vi "Test DeviceManager API.vi"() -> ()   [LabVIEW 2023, in "DeviceManager.lvlib"]
doc: "DeviceManager API Tester."
uses:
  DeviceManager.lvlib
  <vilib>/Utility/error.llb/DialogType.ctl
  2ec88339-7153-484d-8eb7-3b0f2fceeaf8.vi
  SCD/SCD.lvclass
  Mono/Monochromator.lvclass
  CCD/CCD.lvclass
  <vilib>/JDP Science/JSONtext/Variant to JSON Text.vi
  <vilib>/JDP Science/JSONtext/LVClass Serializer/JSONtext LVClass Serializer.lvclass
  <vilib>/Hampel Software Engineering/HSE Logger/hse-logger.lvlib
panel:
  in  "DevicesList":bool
  in  "DiscoverDevices":bool
  in  "JSON to be sent":string="{\"id\":1234, \"command\":\"icl_info\"}"
  in  "SendJSONandAskForReply":bool
  in  "ICLshutdown":bool
  in  "WS Server Port":string="25010"
  in  "WS Server IP":string="ws://127.0.0.1"
  in  "OpenWebSocketCommunication":bool
  in  "StartICL":bool
  out "last error":errorcluster
  in  "Show Diagram on Init":bool
  in  "Show Block Diagram":bool
  in  "Stop Module":bool
  in  "Start Module":bool
  in  "Hide Module Panel":bool
  in  "Show Module Panel":bool
  out "Status":string
  out "Module Running?":bool
  # "This VI tests the API for the Module."
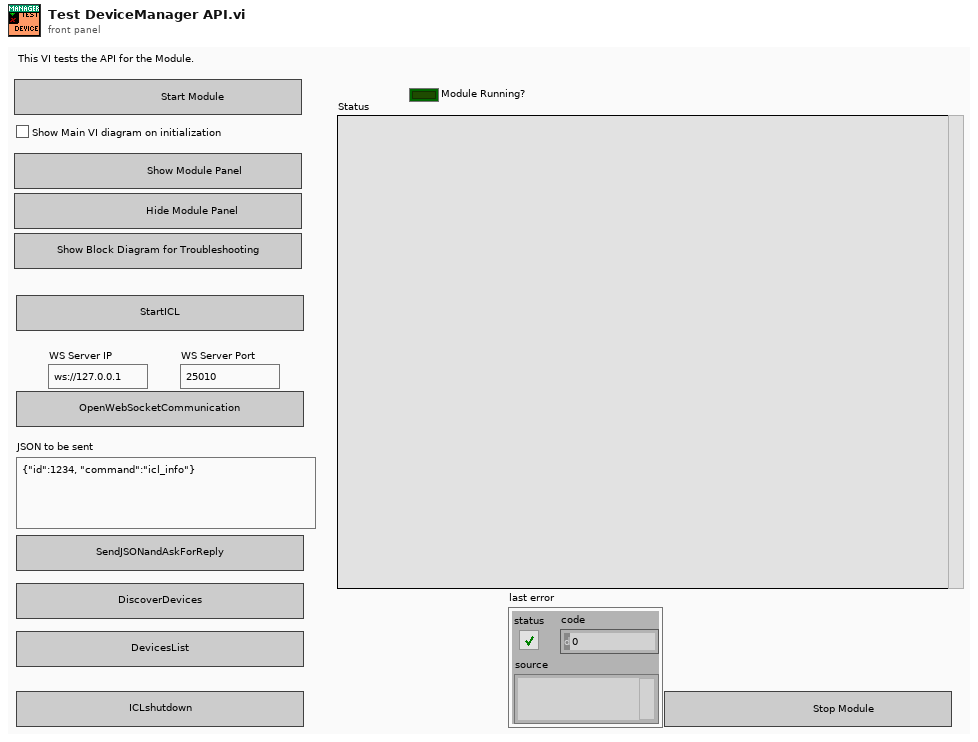
[diagram p1: front panel]
types:
  T1 = typedef "DeviceManager.lvlib/Broadcast Events--cluster.ctl" = cluster{"Module Did Init":refnum<user-event>, "Status Updated":refnum<user-event>, "Error Reported":refnum<user-event>, "Module Did Stop":refnum<user-event>, "Update Module Execution Status":refnum<user-event>}
  T2 = typedef "DialogType.ctl" = u16
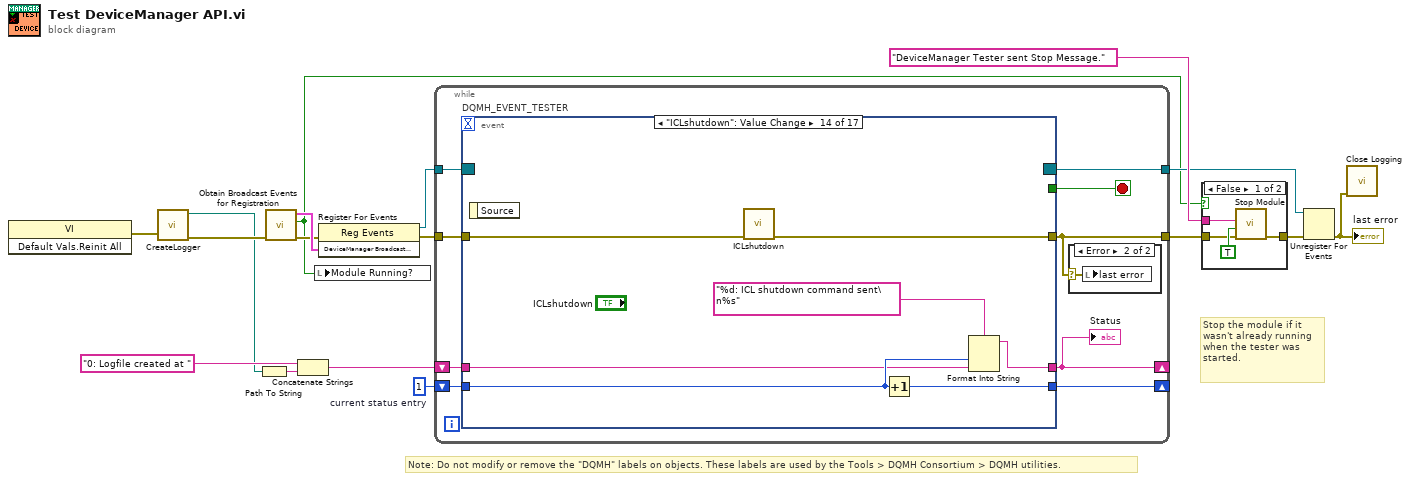
[diagram p0: block diagram]
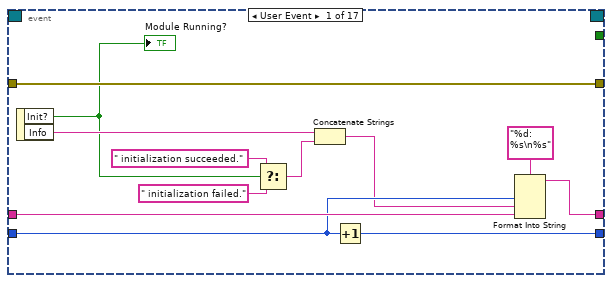
[diagram p4: hidden frame]
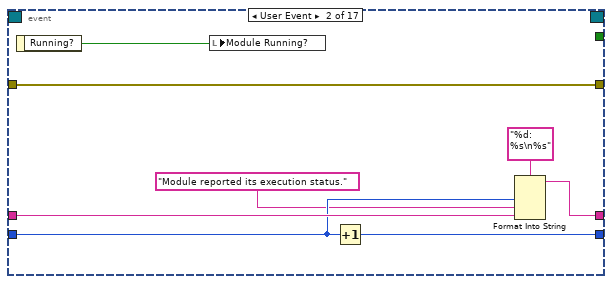
[diagram p5: hidden frame]
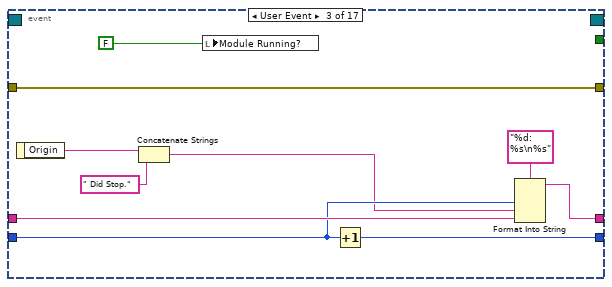
[diagram p6: hidden frame]
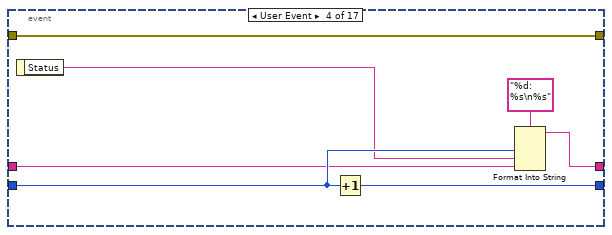
[diagram p7: hidden frame]
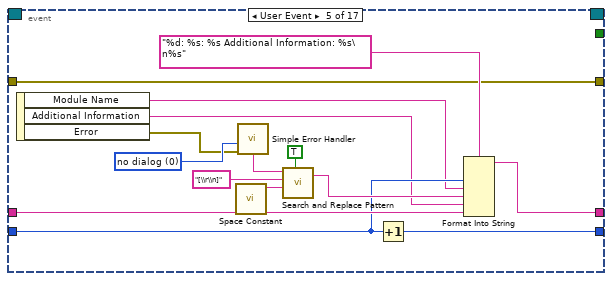
[diagram p8: hidden frame]
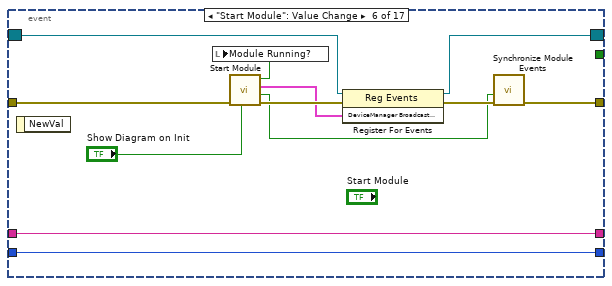
[diagram p9: hidden frame]
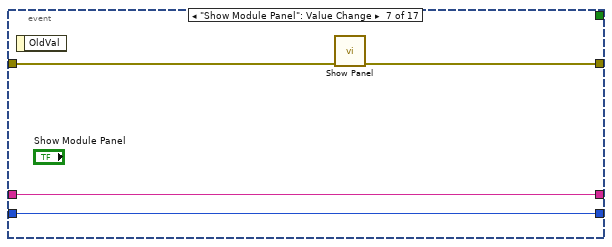
[diagram p10: hidden frame]
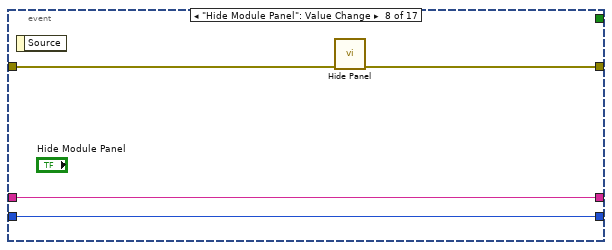
[diagram p11: hidden frame]
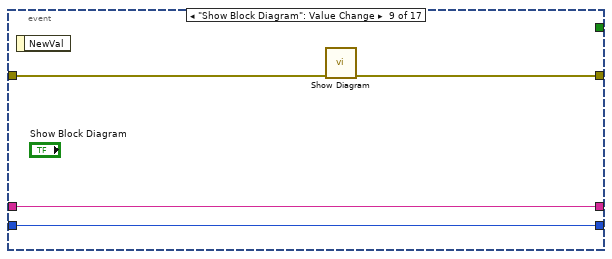
[diagram p12: hidden frame]
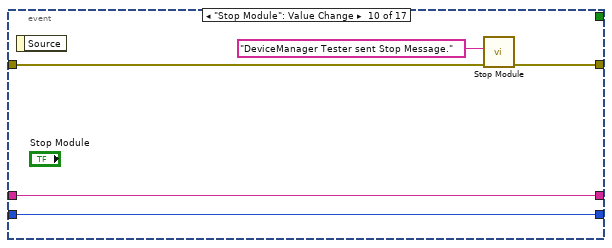
[diagram p13: hidden frame]
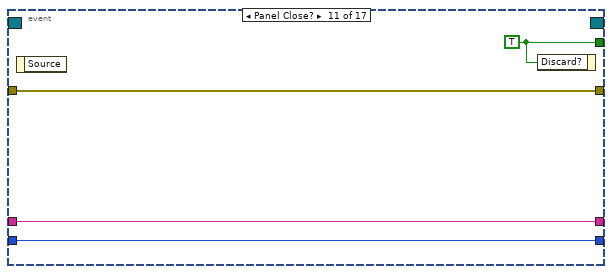
[diagram p14: hidden frame]
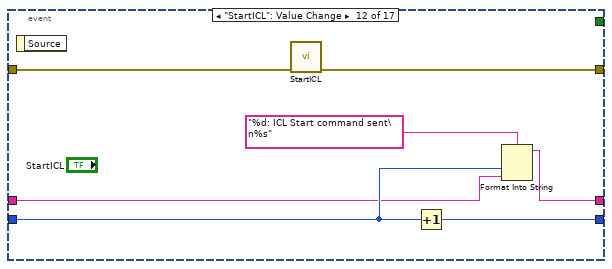
[diagram p15: hidden frame]
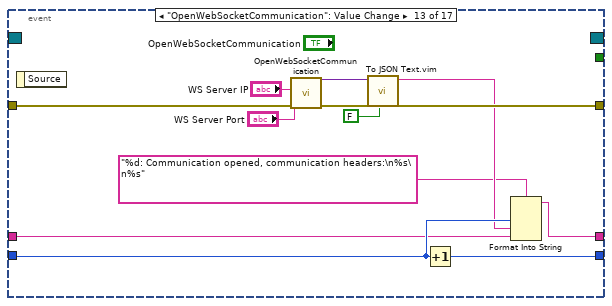
[diagram p16: hidden frame]
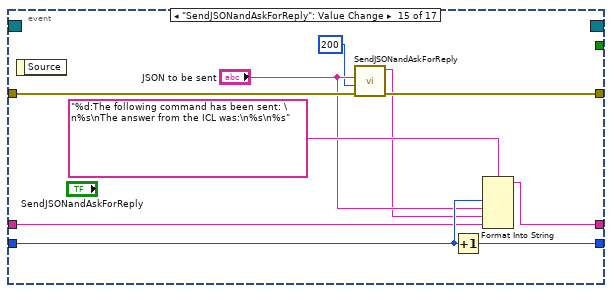
[diagram p17: hidden frame]
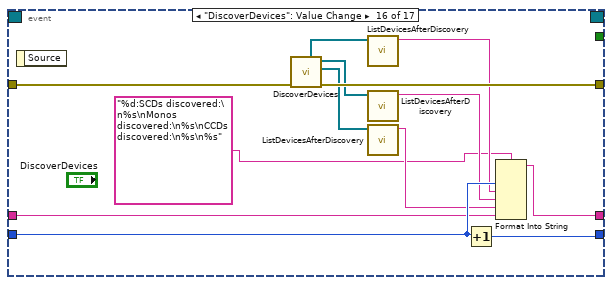
[diagram p18: hidden frame]
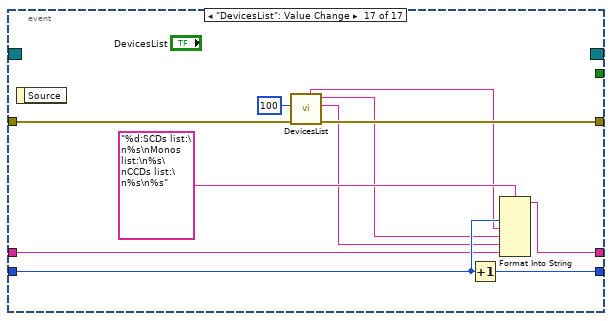
[diagram p19: hidden frame]
diagram:
  w15 = 1  # current status entry
  # "Stop the module if it wasn't already running when the tester was started."
  # "Note: Do not modify or remove the \"DQMH\" labels on objects. These labels are used by the Tools > DQMH Consortium > DQMH utilities."
  n1 = invoke class="VI" method="Default Vals.Reinit All"() -> (error out=w7:errorcluster)  [unwired: 3 in, 2 out]
  n2 = call "CreateLogger.vi"("error in (no error)"=w7) -> ("error out"=w6:errorcluster, "log-file path"=w4:path)  [unwired: 9 in]
  n3 = Path To String(path=w4) -> (string=w3:string)
  n4 = call "Obtain Broadcast Events for Registration.vi"("error in"=w6) -> ("error out"=w10:errorcluster, "Already running?"=w9:bool, "DeviceManager Broadcast Events"=w13:T1)  [unwired: 8 in]
  n5 = Concatenate Strings("0: Logfile created at " ("string"), w3) -> (w2:string)
  n6 = local write "Module Running?"(w9) -> ()
  n7 = register-events(error in=w10, w13) -> (reference out=w12:refnum<event-registration>, error out=w14:errorcluster)  [unwired: 1 in]
  n8 = while {
    tunnel: w12 -> [w26]
    tunnel: [w18] -> w8
    shift-right: [w22] -> _
    shift-left: w2 -> [w24]
    shift-right: [w23] -> _
    shift-left: w15 -> [w25]
    tunnel: w14 -> [w21]
    tunnel: [w20] -> w11
    stop <- w19 stop-if-true
    n9 = event "DQMH_EVENT_TESTER" shown="[13] \"ICLshutdown\": Value Change" {
      selector: w26 -> [_ _ _ _ _ w85 _ _ _ _ _ _ _ _ _ _ _]
      dyn-events: [_ _ _ _ _ w84 _ _ _ _ _ _ _ _ _ _ _] -> w20
      timeout: _ -> [_ _ _ _ _ _ _ _ _ _ _ _ _ _ _ _ _]
      tunnel: [_ _ _ _ _ _ _ _ _ _ w112 _ _ _ _ _ _] -> w19
      tunnel: [w39 w41 w48 w58 w68 w83 w95 w99 w100 w106 w109 w118 w130 w137 w147 w160 w171] -> w18
      tunnel: w25 -> [w36 w45 w55 w61 w71 w88 w93 w97 w101 w107 w110 w117 w126 w135 w145 w159 w168]
      tunnel: w24 -> [w37 w46 w56 w60 w72 w89 w94 w98 w102 w108 w111 w115 w123 w133 w141 w155 w165]
      tunnel: [w34 w43 w53 w62 w70 w89 w94 w98 w102 w108 w111 w114 w122 w134 w143 w149 w166] -> w22
      tunnel: [w35 w44 w54 w64 w69 w88 w93 w97 w101 w107 w110 w116 w127 w136 w146 w158 w167] -> w23
      tunnel: w21 -> [w39 w41 w48 w58 w68 w82 w92 w96 w103 w104 w109 w119 w131 w138 w148 w161 w172]
      event User Event {
        n10 = event-data() -> ("Init?"=w31:bool, "Info"=w33:string)  [unwired: 1 in]
        "Module Running?" <- w31
        n11 = Select(t=" initialization succeeded.", s=w31, f=" initialization failed.") -> (s? t:f=w28:string)
        n12 = Concatenate Strings(w33, w28) -> (w32:string)
        n13 = Increment(x=w36) -> (x+1=w35:i32)
        n14 = Format Into String(format string="%d: %s\n%s", w36, w32, w37) -> (resulting string=w34:string)  [unwired: 2 in, 1 out]
      }
      event User Event {
        n15 = event-data() -> ("Running?"=w40:bool)  [unwired: 1 in]
        n16 = local write "Module Running?"(w40) -> ()
        n17 = Increment(x=w45) -> (x+1=w44:i32)
        n18 = Format Into String(format string="%d: %s\n%s", w45, "Module reported its execution status.", w46) -> (resulting string=w43:string)  [unwired: 2 in, 1 out]
      }
      event User Event {
        n19 = event-data() -> ("Origin"=w52:string)  [unwired: 1 in]
        n20 = Concatenate Strings(w52, " Did Stop.") -> (w51:string)
        n21 = local write "Module Running?"(FALSE ("Module Did Init?")) -> ()
        n22 = Increment(x=w55) -> (x+1=w54:i32)
        n23 = Format Into String(format string="%d: %s\n%s", w55, w51, w56) -> (resulting string=w53:string)  [unwired: 2 in, 1 out]
      }
      event User Event {
        n24 = event-data() -> ("Status"=w59:string)  [unwired: 1 in]
        n25 = Increment(x=w61) -> (x+1=w64:i32)
        n26 = Format Into String(format string="%d: %s\n%s", w61, w59, w60) -> (resulting string=w62:string)  [unwired: 2 in, 1 out]
      }
      event User Event {
        w73 = T2 0 items=["no dialog", "OK message", "continue or stop message", "OK message + warnings", "continue/stop + warnings"] ("type of dialog (OK msg:1)")
        n27 = event-data() -> ("Module Name"=w67:string, "Additional Information"=w66:string, "Error"=w65:errorcluster)  [unwired: 1 in]
        n28 = call <vilib>:"Space Constant.vi"() -> ("String"=w77:string)
        n29 = call <vilib>:"Simple Error Handler.vi"("type of dialog (OK msg:1)"=w73, "error in (no error)"=w65) -> ("message"=w74:string)  [unwired: 3 in, 4 out]
        n30 = call <vilib>:"Search and Replace Pattern.vi"("string"=w74, "regular expression (\"\")"="[\\r\\n]" ("regular expression (\"\")"), "replace string (\"\")"=w77, "replace all? (F)"=TRUE ("replace all CR/LF with spaces")) -> ("result string"=w75:string)  [unwired: 1 in, 1 out]
        n31 = Increment(x=w71) -> (x+1=w69:i32)
        n32 = Format Into String(format string="%d: %s: %s Additional Information: %s\n%s", w71, w67, w75, w66, w72) -> (resulting string=w70:string)  [unwired: 2 in, 1 out]
      }
      event "Start Module": Value Change {
        n33 = event-data() -> ()  [unwired: 1 in, 1 out]
        n34 = call "Start Module.vi"("Show Main VI Diagram on Init (F)"="Show Diagram on Init", "error in"=w82) -> ("error out"=w90:errorcluster, "Wait for Event Sync?"=w87:bool, "DeviceManager Broadcast Events"=w86:T1, "Module Was Already Running?"=w81:bool)  [unwired: 6 in]
        n35 = local write "Module Running?"(w81) -> ()
        n36 = register-events(reference=w85, error in=w90, w86) -> (reference out=w84:refnum<event-registration>, error out=w91:errorcluster)
        n37 = call "Synchronize Module Events.vi"("error in"=w91, "Wait for Event Sync?"=w87) -> ("error out"=w83:errorcluster)  [unwired: 9 in]
      }
      event "Show Module Panel": Value Change {
        n38 = event-data() -> ()  [unwired: 1 in, 1 out]
        n39 = call "Show Panel.vi"("error in"=w92) -> ("error out"=w95:errorcluster)  [unwired: 10 in]
      }
      event "Hide Module Panel": Value Change {
        n40 = event-data() -> ()  [unwired: 1 in, 1 out]
        n41 = call "Hide Panel.vi"("error in"=w96) -> ("error out"=w99:errorcluster)  [unwired: 10 in]
      }
      event "Show Block Diagram": Value Change {
        n42 = event-data() -> ()  [unwired: 1 in, 1 out]
        n43 = call "Show Diagram.vi"("error in"=w103) -> ("error out"=w100:errorcluster)  [unwired: 10 in]
      }
      event "Stop Module": Value Change {
        n44 = event-data() -> ()  [unwired: 1 in, 1 out]
        n45 = call "Stop Module.vi"("error in"=w104, "Origin"="DeviceManager Tester sent Stop Message.") -> ("error out"=w106:errorcluster)  [unwired: 9 in]
      }
      event Panel Close? {
        w112 = TRUE ("Discard?")
        n46 = event-data() -> ()  [unwired: 1 in, 1 out]
        n47 = event-data("Discard?"=w112) -> ()  [unwired: 1 in, 1 out]
      }
      event "StartICL": Value Change {
        n48 = event-data() -> ()  [unwired: 1 in, 1 out]
        n49 = call "StartICL.vi"("error in"=w119) -> ("error out"=w118:errorcluster)  [unwired: 10 in]
        n50 = Increment(x=w117) -> (x+1=w116:i32)
        n51 = Format Into String(format string="%d: ICL Start command sent\n%s", w117, w115) -> (resulting string=w114:string)  [unwired: 2 in, 1 out]
      }
      event "OpenWebSocketCommunication": Value Change {
        n52 = event-data() -> ()  [unwired: 1 in, 1 out]
        n53 = call "OpenWebSocketCommunication.vi"("error in"=w131, "WS Server Port"="WS Server Port", "WS Server IP"="WS Server IP") -> ("error out"=w130:errorcluster, "Return Headers"=w125:variant)  [unwired: 6 in, 1 out]
        n54 = call "To JSON Text.vim"("Pretty Print?"=FALSE, "Anything"=w125) -> ("<JSON>"=w121:string)  [unwired: 8 in, 1 out]
        n55 = Increment(x=w126) -> (x+1=w127:i32)
        n56 = Format Into String(format string="%d: Communication opened, communication headers:\n%s\n%s", w126, w121, w123) -> (resulting string=w122:string)  [unwired: 2 in, 1 out]
      }
      event "ICLshutdown": Value Change {
        n57 = event-data() -> ()  [unwired: 1 in, 1 out]
        n58 = call "ICLshutdown.vi"("error in"=w138) -> ("error out"=w137:errorcluster)  [unwired: 10 in]
        n59 = Increment(x=w135) -> (x+1=w136:i32)
        n60 = Format Into String(format string="%d: ICL shutdown command sent\n%s", w135, w133) -> (resulting string=w134:string)  [unwired: 2 in, 1 out]
      }
      event "SendJSONandAskForReply": Value Change {
        n61 = event-data() -> ()  [unwired: 1 in, 1 out]
        n62 = call "SendJSONandAskForReply.vi"("error in"=w148, "Delay between send and receive [ms]"=200, "JSON to be sent"="JSON to be sent") -> ("error out"=w147:errorcluster, "JSON reply"=w140:string)  [unwired: 6 in, 1 out]
        n63 = Increment(x=w145) -> (x+1=w146:i32)
        n64 = Format Into String(format string="%d:The following command has been sent: \n%s\nThe answer from the ICL was:\n%s\n%s", w145, "JSON to be sent", w140, w141) -> (resulting string=w143:string)  [unwired: 2 in, 1 out]
      }
      event "DiscoverDevices": Value Change {
        n65 = event-data() -> ()  [unwired: 1 in, 1 out]
        n66 = call "DiscoverDevices.vi"("error in"=w161) -> ("error out"=w160:errorcluster, "CCDs"=w153:refnum<class "CCD.lvclass">[], "Monos"=w154:refnum<class "Monochromator.lvclass">[], "SCDs"=w157:refnum<class "SCD.lvclass">[])  [unwired: 6 in, 1 out]
        n67 = call "ListDevicesAfterDiscovery.vi"("SCDs"=w157) -> ("List of devices"=w156:string)  [unwired: 10 in]
        n68 = call "ListDevicesAfterDiscovery.vi"("SCDs"=w154) -> ("List of devices"=w152:string)  [unwired: 10 in]
        n69 = call "ListDevicesAfterDiscovery.vi"("SCDs"=w153) -> ("List of devices"=w151:string)  [unwired: 10 in]
        n70 = Increment(x=w159) -> (x+1=w158:i32)
        n71 = Format Into String(format string="%d:SCDs discovered:\n%s\nMonos discovered:\n%s\nCCDs discovered:\n%s\n%s", w159, w156, w152, w151, w155) -> (resulting string=w149:string)  [unwired: 2 in, 1 out]
      }
      event "DevicesList": Value Change {
        n72 = event-data() -> ()  [unwired: 1 in, 1 out]
        n73 = call "DevicesList.vi"("error in"=w172, "Time out [ms]"=100) -> ("error out"=w171:errorcluster, "CCD-results"=w162:string, "monochromator results"=w163:string, "SCD-results"=w164:string)  [unwired: 5 in, 1 out]
        n74 = Increment(x=w168) -> (x+1=w167:i32)
        n75 = Format Into String(format string="%d:SCDs list:\n%s\nMonos list:\n%s\nCCDs list:\n%s\n%s", w168, w164, w163, w162, w165) -> (resulting string=w166:string)  [unwired: 2 in, 1 out]
      }
    }
    "Status" <- w22
    n76 = case shown="Error" w18 {
      selector: w18 -> [_ w27]
      frame No Error {
      }
      frame Error {
        n77 = local write "last error"(w27) -> ()
      }
    }
  }
  n78 = case shown="False" w9 {
    tunnel: [w176 w177] -> w17
    tunnel: "DeviceManager Tester sent Stop Message." ("Origin") -> [w175 _]
    tunnel: w8 -> [w173 w177]
    frame False {
      n79 = call "Stop Module.vi"("error in"=w173, "Wait for Module to Stop? (F)"=TRUE ("Wait for Module to stop?"), "Origin"=w175) -> ("error out"=w176:errorcluster)  [unwired: 8 in]
    }
    frame True {
    }
  }
  n80 = Unregister For Events(event registration refnum=w11, error in=w17) -> (error out=w1:errorcluster)
  "last error" <- w1
  n81 = call <vilib>:"Close Logging.vi"("error in"=w1) -> ()  [unwired: 10 in, 1 out]
